vi "Path Parameter SLM.vi"(2 "Action":u16(ring) items=["ParamAuto", "ParamUser"]) -> (10 "appended path":path)   [LabVIEW 2012]
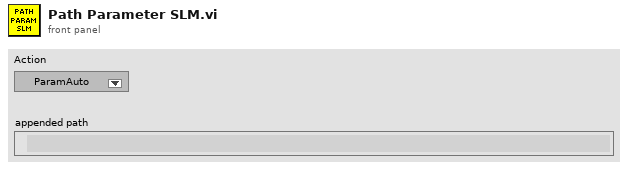
[diagram p1: front panel]
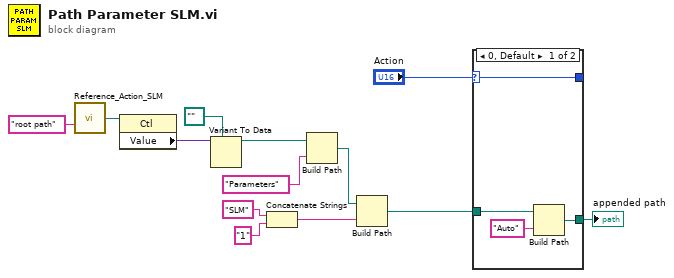
[diagram p0: block diagram]
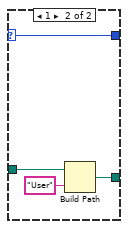
[diagram p2: hidden frame]
diagram:
  n1 = call "Reference_Action_SLM.vi"("Control Name"="root path") -> ("Ref OUT"=w4:refnum<vi>)  [unwired: 12 in, 2 out]
  n2 = property class="Ctl"(reference=w4) -> ("Value"=w3:variant)  [unwired: 1 in, 2 out]
  n3 = Variant To Data(type=path "" ("Path"), Variant=w3) -> (data=w1:path)  [unwired: 1 in, 1 out]
  n4 = Concatenate Strings("SLM" ("name or relative path"), "1" ("string")) -> (w9:string)
  n5 = Build Path(base path=w1, name or relative path="Parameters") -> (appended path=w12:path)
  n6 = Build Path(base path=w12, name or relative path=w9) -> (appended path=w8:path)
  n7 = case shown="0, Default" "Action" {
    selector: "Action" -> [w14 w18]
    tunnel: w8 -> [w16 w21]
    tunnel: [w15 w20] -> w6
    tunnel: [w14 w18] -> _
    frame 0, Default {
      n8 = Build Path(base path=w16, name or relative path="Auto") -> (appended path=w15:path)
    }
    frame 1 {
      n9 = Build Path(base path=w21, name or relative path="User") -> (appended path=w20:path)
    }
  }
  "appended path" <- w6
